vi "cw_4_6.vi"() -> ()   [LabVIEW 2022 SP3]
panel:
  out "number of occurances":i32
  in  "what to look for?":string
  in  "String":string
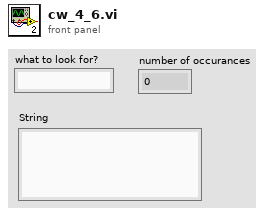
[diagram p1: front panel]
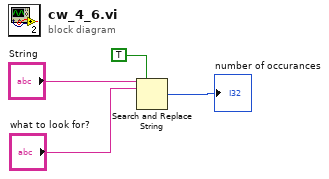
[diagram p0: block diagram]
diagram:
  n1 = Search and Replace String(replace all?=TRUE ("replace all? (F)"), input string="String", search string="what to look for?") -> (number of replacements=→"number of occurances":i32)  [unwired: 5 in, 3 out]
